vi "Lambda_Configuration.vi"() -> ()   [LabVIEW 2015]
uses:
  <vilib>/Utility/error.llb/DialogType.ctl
panel:
  out "Output Current":dbl format="%.4f"
  out "Output Voltage":dbl format="%.4f"
  out "Response":string
  out "Serial Number:":string
  out "error?":bool
  out "Model:":string
  in  "Reset (T)":bool=TRUE
  in  "BAUD":u16(ring)=3 items=["1200", "2400", "4800", "9600", "19200"]
  in  "GEN Addr":i16=6
  in  "VISA name":refnum<visa-resource-name>
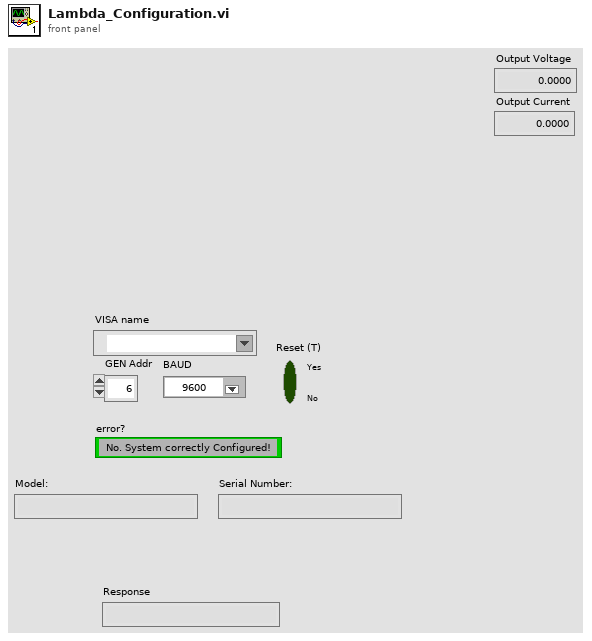
[diagram p1: front panel]
types:
  T1 = typedef "DialogType.ctl" = u16
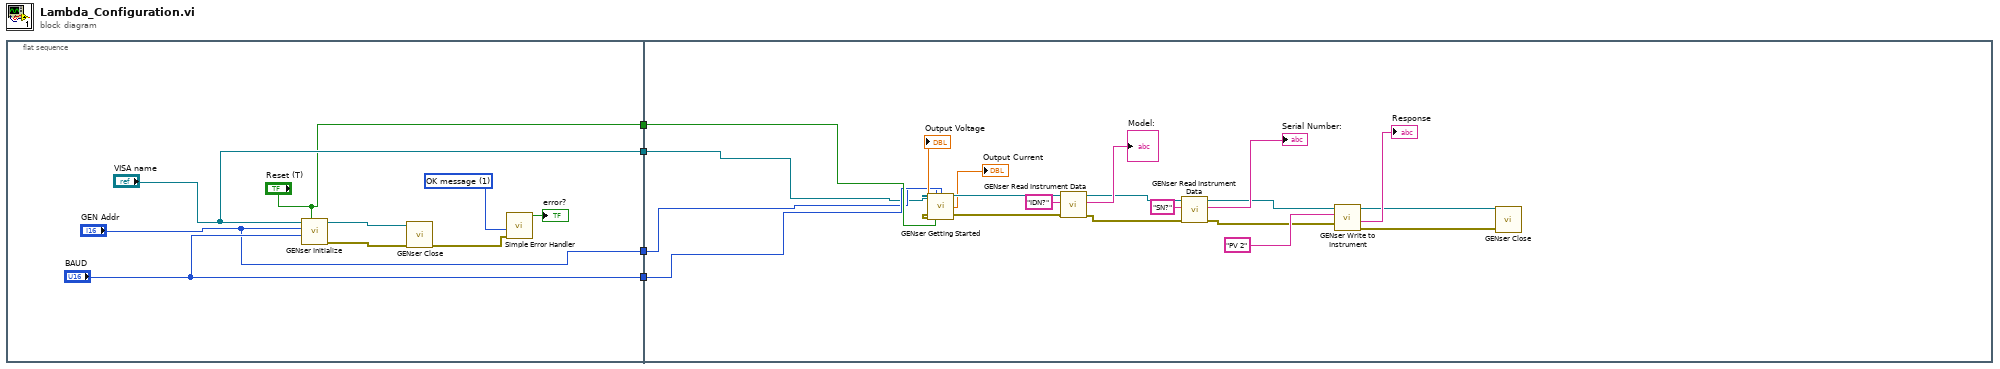
[diagram p0: block diagram]
diagram:
  n1 = flat-sequence {
    tunnel: ["BAUD"] -> w4
    tunnel: ["GEN Addr"] -> w3
    tunnel: ["VISA name"] -> w2
    tunnel: ["Reset (T)"] -> w1
    tunnel: w4 -> [w16]
    tunnel: w3 -> [w15]
    tunnel: w2 -> [w14]
    tunnel: w1 -> [w17]
    frame #0 {
      w10 = T1 1 items=["no dialog", "OK message", "continue or stop message", "OK message + warnings", "continue/stop + warnings"] ("type of dialog (OK msg:1)")
      n2 = call <instrlib>:"GENser Initialize.vi"("Reset (T)"="Reset (T)", "BAUD"="BAUD", "GEN Addr"="GEN Addr", "VISA name"="VISA name") -> ("error out"=w12:errorcluster, "VISA out"=w13:refnum<visa-resource-name>)  [unwired: 6 in]
      n3 = call <instrlib>:"GENser Close.vi"("error"=w12, "VISA name"=w13) -> ("error out"=w11:errorcluster)  [unwired: 9 in]
      n4 = call <vilib>:"Simple Error Handler.vi"("type of dialog (OK msg:1)"=w10, "error in (no error)"=w11) -> ("error?"=→"error?":bool)  [unwired: 3 in, 4 out]
    }
    frame #1 {
      n5 = call <instrlib>:"GENser Getting Started.vi"("VISA"=w14, "GEN Addr"=w15, "BAUD"=w16, "Reset (T)"=w17) -> ("VISA out"=w23:refnum<visa-resource-name>, "Output Voltage"=→"Output Voltage":dbl, "Output Current"=→"Output Current":dbl, "error out"=w22:errorcluster)  [unwired: 8 in]
      n6 = call <instrlib>:"GENser Read Instrument Data.vi"("error"=w22, "Query"="IDN?", "VISA"=w23) -> ("error out"=w30:errorcluster, "Response"=→"Model:":string, "VISA out"=w31:refnum<visa-resource-name>)  [unwired: 5 in, 1 out]
      n7 = call <instrlib>:"GENser Read Instrument Data.vi"("error"=w30, "Query"="SN?", "VISA"=w31) -> ("error out"=w25:errorcluster, "Response"=→"Serial Number:":string, "VISA out"=w27:refnum<visa-resource-name>)  [unwired: 5 in, 1 out]
      n8 = call <instrlib>:"GENser Write to Instrument.vi"("error"=w25, "Command"="PV 2", "VISA"=w27) -> ("error out"=w18:errorcluster, "Response"=→"Response":string, "VISA out"=w19:refnum<visa-resource-name>)  [unwired: 6 in]
      n9 = call <instrlib>:"GENser Close.vi"("error"=w18, "VISA name"=w19) -> ()  [unwired: 9 in, 1 out]
    }
  }
